vi "createStepMotorFrame.vi"(8 "error in (no error)":errorcluster, 9 "TriggerIRQ":bool, 10 "WaitForTrigger":bool, 11 "HardPointActuator in":refnum<class "HPILC.lvclass">) -> (0 "error out":errorcluster, 2 "Frame":T1 {"Data" format="%02x"}, 3 "HardPointActuator out":refnum<class "HPILC.lvclass">)   [LabVIEW 2016, in "RTHPILC.lvlib" / "HPILC.lvclass"]
uses:
  HPILC.lvclass
  D:/Code/Common_RT_ILC/ILC/ILC.lvclass
  Common_RT_Modbus/DataTypes/Frame.ctl
  Common_RT_Modbus/DynamicFrameBuilder/DynamicFrameBuilder.lvclass
  HPILC.lvclass/HPILC.ctl
  Common_RT_ILC/ILC/ILC.lvclass/ILC.ctl
  Common_RT_ILC/ILC/ILC.lvclass
  Common_RT_Modbus/RTModbus.lvlib
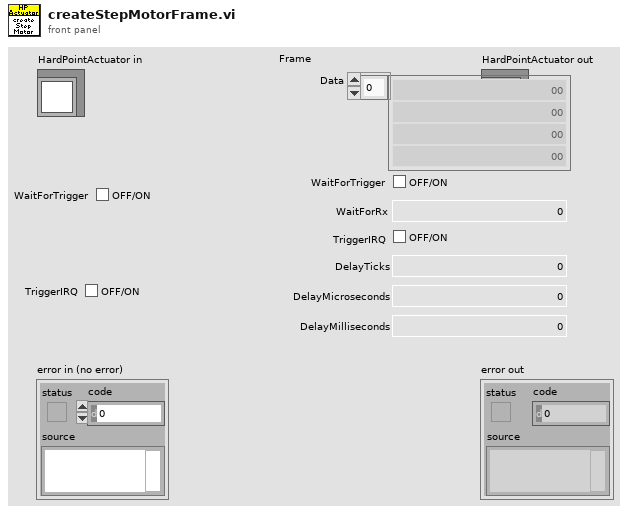
[diagram p1: front panel]
types:
  T1 = typedef "RTModbus.lvlib/Frame.ctl" = cluster{"Data":u8[], "WaitForTrigger":bool, "WaitForRx":u16, "TriggerIRQ":bool, "DelayTicks":u16, "DelayMicroseconds":u16, "DelayMilliseconds":u16}
  T2 = typedef "RTILC.lvlib/ILCData.ctl" = cluster{"Constants":T3, "Command":T4, "Telemetry":T6, "Responses":T7, "Timings":T9}
  T3 = typedef "RTILC.lvlib/ILCConstants.ctl" = cluster{"Subnet":u8, "Address":u8}
  T4 = typedef "RTILC.lvlib/ILCCommand.ctl" = cluster{"ILCMode":u16, "TemporaryAddress":u8, "ADCScanRate":T5, "ADCChannel":u8, "ADCOffset":sgl, "ADCSensitivity":sgl}
  T5 = typedef "RTILC.lvlib/ILCScanRates.ctl" = u8
  T6 = typedef "RTILC.lvlib/ILCTelemetry.ctl" = cluster{"UniqueID":u64, "FirmwareType":u8, "NetworkNodeType":u8, "ILCOption":u8, "NetworkNodeOption":u8, "MajorRevision":u8, "MinorRevision":u8, "FirmwareName":string, "ILCMode":u16, "MajorFault":bool, "MinorFault":bool, "FaultOverride":bool, "UniqueIDCRCMismatch":bool, "AppTypeNodeTypeMismatch":bool, "AppMissing":bool, "AppCRCMismatch":bool, "TEDSNotFound":bool, "TEDS1Mismatch":bool, "TEDS2Mismatch":bool, "WatchdogResetDetected":bool, "BrownoutDetected":bool, "EventTrapResetDetected":bool, "TemporaryAddress":u8, "ADCScanRate":T5, "DAC1":u16, "DAC2":u16, "DAC3":u16, "DAC4":u16, "MainADCCalibrationK":sgl[], "MainSensorOffset":sgl[], "MainSensorSensitivity":sgl[], "BackupADCCalibrationK":sgl[], "BackupSensorOffset":sgl[], "BackupSensorSensitivity":sgl[]}
  T7 = typedef "RTILC.lvlib/ILCResponses.ctl" = cluster{"ReportServerID":T8, "ReportServerStatus":T8, "ILCMode":T8, "SetTemporaryAddress":T8, "Reset":T8, "ADCScanRate":T8, "ADCOffsetSensitivity":T8, "ReadDAC":T8, "ReadCalibration":T8}
  T8 = typedef "RTModbus.lvlib/ExceptionCodes.ctl" = u16
  T9 = typedef "RTILC.lvlib/ILCTimings.ctl" = cluster{"ADCOffsetSensitivity":u32, "ADCScanRate":u32, "ILCMode":u32, "ReadCalibration":u32, "ReportServerID":u32, "ReportServerStatus":u32, "Reset":u32, "SetTemporaryAddress":u32}
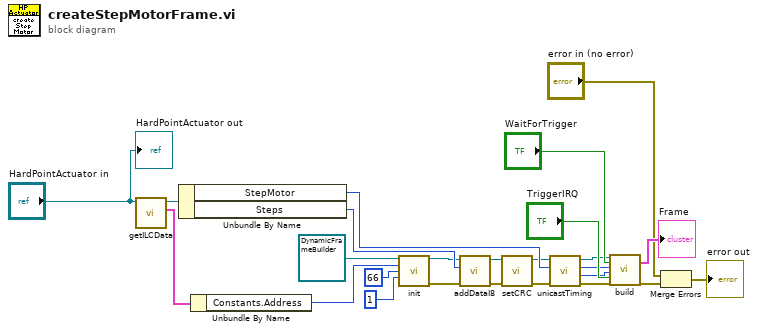
[diagram p0: block diagram]
diagram:
  n1 = call "getILCData.vi"("ILC in"="HardPointActuator in") -> ("ILCData"=w24:T2, "ILC out"=w25:refnum<class "HPILC.lvclass">)  [unwired: 9 in]
  n2 = Unbundle By Name(w25) -> ("StepMotor"=w7:u32, "Steps"=w23:i8)
  n3 = Unbundle By Name(w24) -> ("Constants.Address"=w22:u8)
  n4 = call "init.vi"("DynamicFrameBuilder in"=refnum<class "DynamicFrameBuilder.lvclass"> refnum ("RTModbus.lvlib:DynamicFrameBuilder.lvclass"), "Address"=w22, "Function"=u8 66, "DataSize"=1) -> ("DynamicFrameBuilder out"=w18:refnum<class "DynamicFrameBuilder.lvclass">, "error out"=w19:errorcluster)  [unwired: 10 in]
  n5 = call "addDataI8.vi"("error in (no error)"=w19, "Data"=w23, "DynamicFrameBuilder in"=w18) -> ("error out"=w11:errorcluster, "DynamicFrameBuilder out"=w16:refnum<class "DynamicFrameBuilder.lvclass">)  [unwired: 7 in]
  n6 = call "setCRC.vi"("error in (no error)"=w11, "DynamicFrameBuilder in"=w16) -> ("error out"=w5:errorcluster, "DynamicFrameBuilder out"=w6:refnum<class "DynamicFrameBuilder.lvclass">)  [unwired: 8 in]
  n7 = call "unicastTiming.vi"("error in (no error)"=w5, "Latency in"=w7, "DynamicFrameBuilder in"=w6) -> ("error out"=w1:errorcluster, "WaitForRxTimeout"=w2:u16, "Latency out"=w3:u32, "DynamicFrameBuilder out"=w4:refnum<class "DynamicFrameBuilder.lvclass">)  [unwired: 5 in]
  n8 = call "build.vi"("DynamicFrameBuilder in"=w4, "WaitForTrigger"="WaitForTrigger", "Latency"=w3, "WaitForRxTimeout"=w2, "TriggerIRQ"="TriggerIRQ", "error in (no error)"=w1) -> ("Frame"=→"Frame":T1, "error out"=w14:errorcluster)  [unwired: 11 in, 1 out]
  n9 = Merge Errors("error in (no error)", w14) -> (→"error out":errorcluster)
  "HardPointActuator out" <- "HardPointActuator in"
